vi "Attenuator_DefinePostion.vi"(3 "位置":T1, 5 "电机":T2) -> (1 "PosOut":i32)   [LabVIEW 2018]
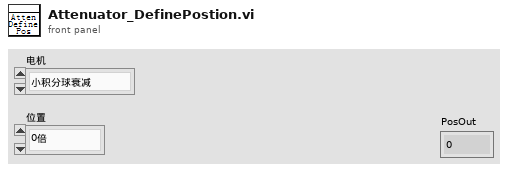
[diagram p1: front panel]
types:
  T1 = typedef "衰减片电机位置枚举器.ctl" = enum16{"0倍", "10倍", "100倍", "1000倍"}
  T2 = typedef "衰减片电机枚举.ctl" = enum16{"小积分球衰减", "偏振仪衰减", "近场相机衰减", "远场相机衰减"}
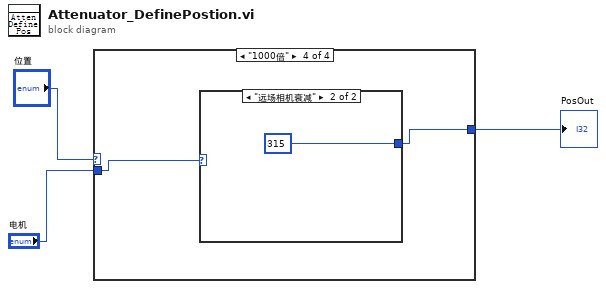
[diagram p0: block diagram]
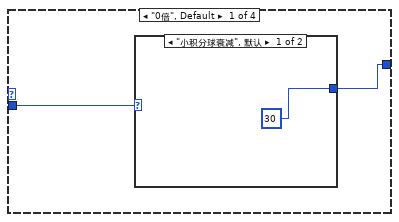
[diagram p2: hidden frame]
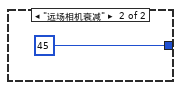
[diagram p3: hidden frame]
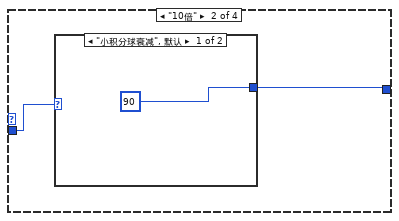
[diagram p4: hidden frame]
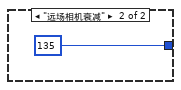
[diagram p5: hidden frame]
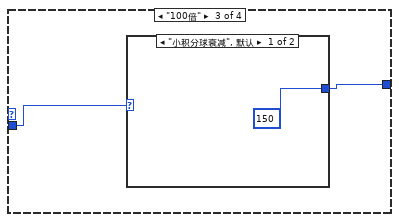
[diagram p6: hidden frame]
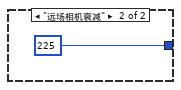
[diagram p7: hidden frame]
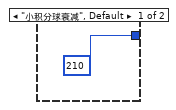
[diagram p8: hidden frame]
diagram:
  n1 = case shown="\"1000倍\"" "位置" {
    tunnel: [w5 w8 w12 w16] -> w2
    tunnel: "电机" -> [w4 w9 w13 w17]
    frame "0倍", Default {
      n2 = case shown="\"小积分球衰减\", 默认" w4 {
        tunnel: [30 45] -> w5
        frame "小积分球衰减", Default {
        }
        frame "远场相机衰减" {
        }
      }
    }
    frame "10倍" {
      n3 = case shown="\"小积分球衰减\", 默认" w9 {
        tunnel: [90 135] -> w8
        frame "小积分球衰减", Default {
        }
        frame "远场相机衰减" {
        }
      }
    }
    frame "100倍" {
      n4 = case shown="\"小积分球衰减\", 默认" w13 {
        tunnel: [150 225] -> w12
        frame "小积分球衰减", Default {
        }
        frame "远场相机衰减" {
        }
      }
    }
    frame "1000倍" {
      n5 = case shown="\"远场相机衰减\"" w17 {
        tunnel: [210 315] -> w16
        frame "小积分球衰减", Default {
        }
        frame "远场相机衰减" {
        }
      }
    }
  }
  "PosOut" <- w2
